vi "Read Data.vi"(8 "error in (no error)":errorcluster, 10 "Count":i32, 11 "VISA Stream in":refnum<class "Serial Stream.lvclass">) -> (0 "error out":errorcluster, 2 "Data":string, 3 "VISA Stream out":refnum<class "Serial Stream.lvclass">)   [LabVIEW 2020, in "Stream-Serial.lvlib" / "Serial Stream.lvclass"]
uses:
  Serial Stream.lvclass
  C:/Program Files (x86)/National Instruments/LabVIEW 2020/vi.lib/IlluminatedG/lv-stream/stream/Stream.lvclass
  Serial Stream.lvclass/Serial Stream.ctl
  <vilib>/IlluminatedG/lv-stream/stream/Stream.lvclass
  C:/dev/IlluminatedG/lv-stream-serial/Stream-Serial/Serial Stream/Serial Stream.lvclass
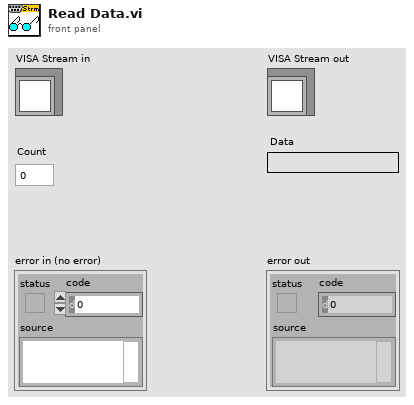
[diagram p1: front panel]
types:
  T1 = typedef "Stream.lvlib/Mode.ctl" = enum16{"Raw", "Buffered", "LineTerm"}
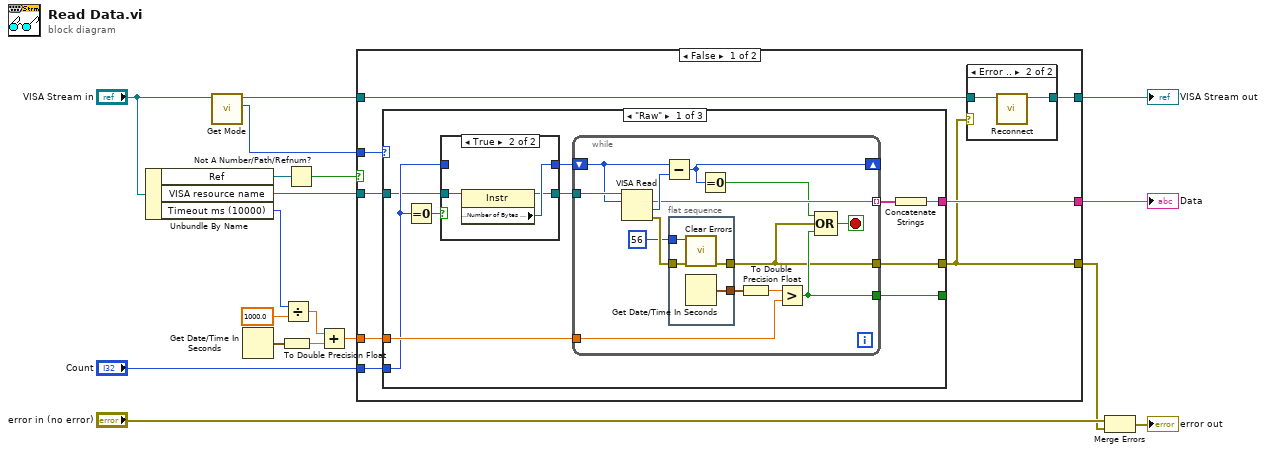
[diagram p0: block diagram]
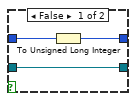
[diagram p2: hidden frame]
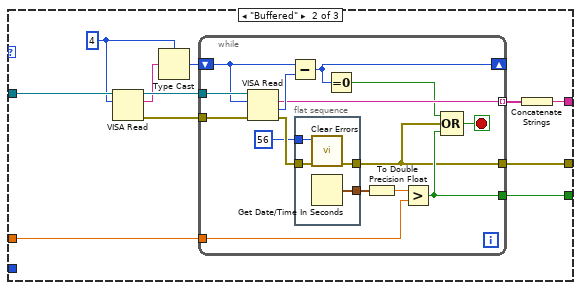
[diagram p3: hidden frame]
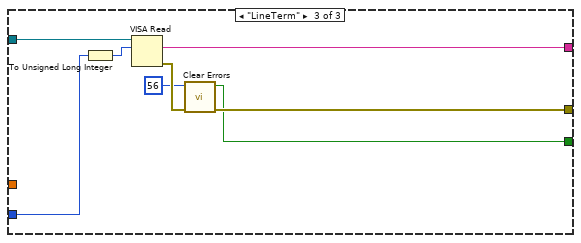
[diagram p4: hidden frame]
diagram:
  n1 = Unbundle By Name("VISA Stream in") -> ("Ref"=w11:refnum<data-value>, "VISA resource name"=w8:refnum<visa-resource-name>, "Timeout ms (10000)"=w12:i32)
  n2 = call <vilib>:"Get Mode.vi"("Stream in"="VISA Stream in") -> ("Mode"=w7:T1, "Stream out"=w6:refnum<class "Serial Stream.lvclass">)  [unwired: 8 in, 1 out]
  n3 = Get Date/Time In Seconds() -> (seconds since 1Jan1904=w17:timestamp)
  n4 = To Double Precision Float(number=w17) -> (double precision float=w15:dbl)
  n5 = Divide(x=w12, y=1000.0) -> (x/y=w14:dbl)
  n6 = Not A Number/Path/Refnum?(number/path/refnum=w11) -> (NaN/Path/Refnum?=w10:bool)
  n7 = Add(x=w14, y=w15) -> (x+y=w9:dbl)
  n8 = case shown="False" w10 {
    tunnel: w9 -> [w24 _]
    tunnel: w8 -> [w26 _]
    tunnel: w7 -> [w25 _]
    tunnel: w6 -> [w21 w102]
    tunnel: "Count" -> [w23 _]
    tunnel: [w22 _] -> w4
    tunnel: [w20 w102] -> w3
    tunnel: [w19 _] -> w1
    frame False {
      n9 = case shown="\"Raw\"" w25 {
        tunnel: w26 -> [w29 w71 w98]
        tunnel: w24 -> [w36 w65 _]
        tunnel: [w33 w64 w91] -> _
        tunnel: [w34 w62 w97] -> w22
        tunnel: w23 -> [w30 _ w96]
        tunnel: [w32 w61 w92] -> w19
        frame "Raw" {
          n10 = Equal To 0?(x=w30) -> (x = 0?=w31:bool)
          n11 = case shown="True" w31 {
            tunnel: w30 -> [w38 _]
            tunnel: w29 -> [w37 w42]
            tunnel: [w39 w41] -> w28
            tunnel: [w37 w40] -> w27
            frame False {
              n12 = To Unsigned Long Integer(number=w38) -> (unsigned 32bit integer=w39:u32)
            }
            frame True {
              n13 = property class="Instr"(reference=w42) -> (reference out=w40:refnum<visa-resource-name>, "Serial Settings:Number of Bytes at Serial Port"=w41:u32)  [unwired: 1 in, 1 out]
            }
          }
          n14 = while {
            tunnel: w27 -> [w56]
            tunnel: w36 -> [w48]
            shift-right: [w47] -> _
            shift-left: w28 -> [w54]
            tunnel: [w53] -> w35 mode=indexing
            tunnel: [w44] -> w33
            tunnel: [w43] -> w32
            stop <- w45 stop-if-true
            n15 = VISA Read(VISA resource name=w56, byte count=w54) -> (read buffer=w53:string, return count=w55:u32, error out=w52:errorcluster)  [unwired: 1 in, 1 out]
            n16 = Subtract(x=w54, y=w55) -> (x-y=w47:u32)
            n17 = flat-sequence {
              tunnel: w52 -> [w60]
              tunnel: 56 ("specific error code to clear (0: all)") -> [w59]
              tunnel: [w58] -> w50
              tunnel: [w57] -> w43
              frame #0 {
                n18 = call <vilib>:"Clear Errors.vi"("error in (no error)"=w60, "specific error code to clear (0: all)"=w59) -> ("error out"=w57:errorcluster)  [unwired: 4 in, 1 out]
                n19 = Get Date/Time In Seconds() -> (seconds since 1Jan1904=w58:timestamp)
              }
            }
            n20 = Equal To 0?(x=w47) -> (x = 0?=w46:bool)
            n21 = To Double Precision Float(number=w50) -> (double precision float=w49:dbl)
            n22 = Greater?(x=w49, y=w48) -> (0:w44:bool)
            n23 = Compound Arithmetic op=OR(w46, w43, w44) -> (w45:bool)
          }
          n24 = Concatenate Strings(w35) -> (w34:string)
        }
        frame "Buffered" {
          w67 = u32 4 ("byte count")
          n25 = VISA Read(VISA resource name=w71, byte count=w67) -> (VISA resource name out=w70:refnum<visa-resource-name>, read buffer=w69:string, error out=w66:errorcluster)  [unwired: 1 in, 1 out]
          n26 = Type Cast(type=w67, x=w69) -> (*(type *) &x=w68:u32)
          n27 = while {
            tunnel: w70 -> [w86]
            tunnel: w66 -> [w85]
            tunnel: w65 -> [w77]
            shift-right: [w76] -> _
            shift-left: w68 -> [w83]
            tunnel: [w82] -> w63 mode=indexing
            tunnel: [w73] -> w64
            tunnel: [w72] -> w61
            stop <- w74 stop-if-true
            n28 = VISA Read(VISA resource name=w86, byte count=w83, error in (no error)=w85) -> (read buffer=w82:string, return count=w84:u32, error out=w81:errorcluster)  [unwired: 1 out]
            n29 = Subtract(x=w83, y=w84) -> (x-y=w76:u32)
            n30 = flat-sequence {
              tunnel: w81 -> [w90]
              tunnel: 56 ("specific error code to clear (0: all)") -> [w89]
              tunnel: [w88] -> w79
              tunnel: [w87] -> w72
              frame #0 {
                n31 = call <vilib>:"Clear Errors.vi"("error in (no error)"=w90, "specific error code to clear (0: all)"=w89) -> ("error out"=w87:errorcluster)  [unwired: 4 in, 1 out]
                n32 = Get Date/Time In Seconds() -> (seconds since 1Jan1904=w88:timestamp)
              }
            }
            n33 = Equal To 0?(x=w76) -> (x = 0?=w75:bool)
            n34 = To Double Precision Float(number=w79) -> (double precision float=w78:dbl)
            n35 = Greater?(x=w78, y=w77) -> (0:w73:bool)
            n36 = Compound Arithmetic op=OR(w75, w72, w73) -> (w74:bool)
          }
          n37 = Concatenate Strings(w63) -> (w62:string)
        }
        frame "LineTerm" {
          n38 = To Unsigned Long Integer(number=w96) -> (unsigned 32bit integer=w95:u32)
          n39 = VISA Read(VISA resource name=w98, byte count=w95) -> (read buffer=w97:string, error out=w94:errorcluster)  [unwired: 1 in, 2 out]
          n40 = call <vilib>:"Clear Errors.vi"("error in (no error)"=w94, "specific error code to clear (0: all)"=56) -> ("error out"=w92:errorcluster, "specific error cleared?"=w91:bool)  [unwired: 4 in]
        }
      }
      n41 = case shown="Error .." w19 {
        tunnel: w21 -> [w99 w101]
        tunnel: [w99 w100] -> w20
        frame No Error {
        }
        frame Error {
          n42 = call "Reconnect.vi"("Serial Stream in"=w101) -> ("Serial Stream out"=w100:refnum<class "Serial Stream.lvclass">)  [unwired: 9 in, 1 out]
        }
      }
    }
    frame True {
      # "#ERROR?"
    }
  }
  "VISA Stream out" <- w3
  "Data" <- w4
  n43 = Merge Errors("error in (no error)", w1) -> (→"error out":errorcluster)
